vi "Lauda Test Program.vi"() -> ()   [LabVIEW 2018, in "Lauda TCU.lvlib"]
uses:
  Lauda TCU.lvlib
  Lauda Settings.ctl
panel:
  out "Running":bool
  out "Connection Error":bool
  in  "stop":bool
  in  "Temp":dbl
  in  "Run":bool
  out "error out":errorcluster
  in  "error in (no error)":errorcluster
  out "Huber Settings":T1
  in  "Huber Settings":T1
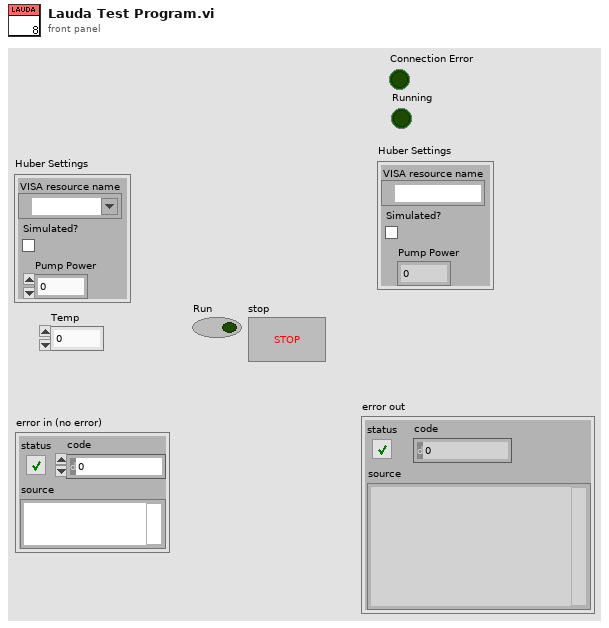
[diagram p1: front panel]
types:
  T1 = typedef "Lauda TCU.lvlib/Lauda Settings.ctl" = cluster{"VISA resource name":refnum<visa-resource-name>, "Simulated?":bool, "Pump Power":i32}
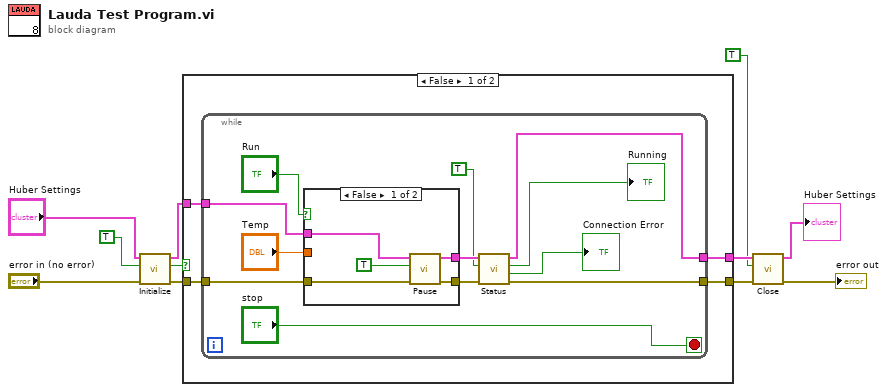
[diagram p0: block diagram]
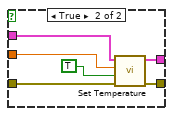
[diagram p2: hidden frame]
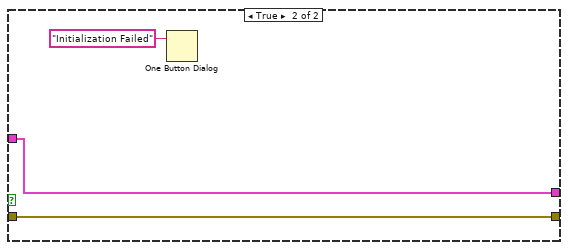
[diagram p3: hidden frame]
diagram:
  n1 = call "Initialize.vi"("error in (no error)"="error in (no error)", "Internal?"=TRUE, "Lauda Settings"="Huber Settings") -> ("error out"=w4:errorcluster, "Connection Error"=w3:bool, "Lauda Settings"=w5:T1)  [unwired: 6 in]
  n2 = case shown="False" w3 {
    tunnel: [w15 w40] -> w9
    tunnel: [w14 w39] -> w7
    tunnel: w5 -> [w13 w40]
    tunnel: w4 -> [w12 w39]
    frame False {
      n3 = while {
        tunnel: [w27] -> w15
        tunnel: [w26] -> w14
        tunnel: w13 -> [w24]
        tunnel: w12 -> [w23]
        stop <- "stop" stop-if-true
        n4 = case shown="False" "Run" {
          tunnel: w24 -> [w32 w38]
          tunnel: w23 -> [w31 w37]
          tunnel: [w30 w36] -> w22
          tunnel: [w29 w35] -> w21
          tunnel: "Temp" -> [_ w34]
          frame False {
            n5 = call "Pause.vi"("error in (no error)"=w31, "Internal?"=TRUE, "Huber Settings"=w32) -> ("error out"=w30:errorcluster, "Huber Settings"=w29:T1)  [unwired: 7 in]
          }
          frame True {
            n6 = call "Set Temperature.vi"("error in (no error)"=w37, "Internal?"=TRUE, "Setpoint"=w34, "Lauda Settings"=w38) -> ("error out"=w36:errorcluster, "Lauda Settings"=w35:T1)  [unwired: 5 in, 1 out]
          }
        }
        n7 = call "Status.vi"("error in (no error)"=w22, "Internal?"=TRUE, "Lauda Settings"=w21) -> ("error out"=w26:errorcluster, "Connection Error"=→"Connection Error":bool, "Running"=→"Running":bool, "Lauda Settings"=w27:T1)  [unwired: 2 in, 3 out]
      }
    }
    frame True {
      n8 = One Button Dialog(message="Initialization Failed") -> ()  [unwired: 1 in, 1 out]
    }
  }
  n9 = call "Close.vi"("error in (no error)"=w7, "Internal?"=TRUE, "Lauda  Settings"=w9) -> ("error out"=→"error out":errorcluster, "Lauda Settings"=→"Huber Settings":T1)  [unwired: 7 in]
